vi "labview_code.vi"() -> ()   [LabVIEW 2025]
uses:
  Program Files (x86)/National Instruments/LabVIEW 2025/examples/Instrument IO/Serial/support/Serial - Settings.ctl
  Program Files (x86)/National Instruments/LabVIEW 2025/examples/Instrument IO/Serial/support/Serial - XON-XOFF Characters.ctl
  Program Files (x86)/National Instruments/LabVIEW 2025/examples/Instrument IO/Serial/support/Serial - ASCII Characters.ctl
  <vilib>/Utility/config.llb/Read Key (U32).vi
  <vilib>/Utility/config.llb/Read Key (String).vi
  <vilib>/Instr/_visa.llb/VISA Configure Serial Port (Instr).vi
  <vilib>/Utility/config.llb/NI_LVConfig.lvlib
panel:
  out "MSG from STM32 board 2":string
  in  "Termination Character 5":u8=10 format="%.0x"
  out "Updated baud rate":string
  out "read buffer 3":string
  in  "Stop 5":bool
  in  "Termination Character 4":u8=10 format="%.0x"
  in  "End Write on Termination Character? 4":bool=TRUE
  in  "XON/XOFF Characters 4":T1={"XON"=enum."DC1", "XOFF"=enum."DC3"}
  in  "Serial Settings 4":T3={"baud rate"=9600, "data bits"=8, "parity"=enum."None", "stop bits"=10, "flow control"=0} {"flow control" items=["None"=0, "XON/XOFF"=1, "RTS/CTS"=2, "DTR/DSR"=4]; "stop bits" items=["1.0"=10, "1.5"=15, "2.0"=20]; "data bits" min=5 max=8 step=1; "baud rate" items=["75"=75, "110"=110, "134"=134, "150"=150, "300"=300, "600"=600, "1200"=1200, "1800"=1800, "2400"=2400, "4800"=4800, "7200"=7200, "9600"=9600, "14400"=14400, "19200"=19200, "28800"=28800, "38400"=38400, "56000"=56000, "57600"=57600, "115200"=115200, "128000"=128000, "230400"=230400]}
  in  "End Read on Termination Character? 4":bool=TRUE
  in  "Stop 4":bool
  in  "Termination Character 3":u8=10 format="%.0x"
  in  "End Write on Termination Character? 3":bool=TRUE
  in  "XON/XOFF Characters 3":T1={"XON"=enum."DC1", "XOFF"=enum."DC3"}
  in  "Serial Settings 3":T3={"baud rate"=9600, "data bits"=8, "parity"=enum."None", "stop bits"=10, "flow control"=0} {"flow control" items=["None"=0, "XON/XOFF"=1, "RTS/CTS"=2, "DTR/DSR"=4]; "stop bits" items=["1.0"=10, "1.5"=15, "2.0"=20]; "data bits" min=5 max=8 step=1; "baud rate" items=["75"=75, "110"=110, "134"=134, "150"=150, "300"=300, "600"=600, "1200"=1200, "1800"=1800, "2400"=2400, "4800"=4800, "7200"=7200, "9600"=9600, "14400"=14400, "19200"=19200, "28800"=28800, "38400"=38400, "56000"=56000, "57600"=57600, "115200"=115200, "128000"=128000, "230400"=230400]}
  in  "End Read on Termination Character? 3":bool=TRUE
  out "read buffer 2":string
  in  "Stop 3":bool
  in  "Termination Character 2":u8=10 format="%.0x"
  in  "End Write on Termination Character? 2":bool=TRUE
  in  "XON/XOFF Characters 2":T1={"XON"=enum."DC1", "XOFF"=enum."DC3"}
  in  "Serial Settings 2":T3={"baud rate"=9600, "data bits"=8, "parity"=enum."None", "stop bits"=10, "flow control"=0} {"flow control" items=["None"=0, "XON/XOFF"=1, "RTS/CTS"=2, "DTR/DSR"=4]; "stop bits" items=["1.0"=10, "1.5"=15, "2.0"=20]; "data bits" min=5 max=8 step=1; "baud rate" items=["75"=75, "110"=110, "134"=134, "150"=150, "300"=300, "600"=600, "1200"=1200, "1800"=1800, "2400"=2400, "4800"=4800, "7200"=7200, "9600"=9600, "14400"=14400, "19200"=19200, "28800"=28800, "38400"=38400, "56000"=56000, "57600"=57600, "115200"=115200, "128000"=128000, "230400"=230400]}
  in  "End Read on Termination Character? 2":bool=TRUE
  out "Data Shift":string
  out "Handshake":string
  out "data out 2":string
  out "read buffer":string
  in  "Stop 2":bool
  in  "Termination Character":u8=10 format="%.0x"
  in  "End Write on Termination Character?":bool=TRUE
  in  "XON/XOFF Characters":T1={"XON"=enum."DC1", "XOFF"=enum."DC3"}
  in  "Serial Settings":T3={"baud rate"=9600, "data bits"=8, "parity"=enum."None", "stop bits"=10, "flow control"=0} {"flow control" items=["None"=0, "XON/XOFF"=1, "RTS/CTS"=2, "DTR/DSR"=4]; "stop bits" items=["1.0"=10, "1.5"=15, "2.0"=20]; "data bits" min=5 max=8 step=1; "baud rate" items=["75"=75, "110"=110, "134"=134, "150"=150, "300"=300, "600"=600, "1200"=1200, "1800"=1800, "2400"=2400, "4800"=4800, "7200"=7200, "9600"=9600, "14400"=14400, "19200"=19200, "28800"=28800, "38400"=38400, "56000"=56000, "57600"=57600, "115200"=115200, "128000"=128000, "230400"=230400]}
  in  "End Read on Termination Character?":bool=TRUE
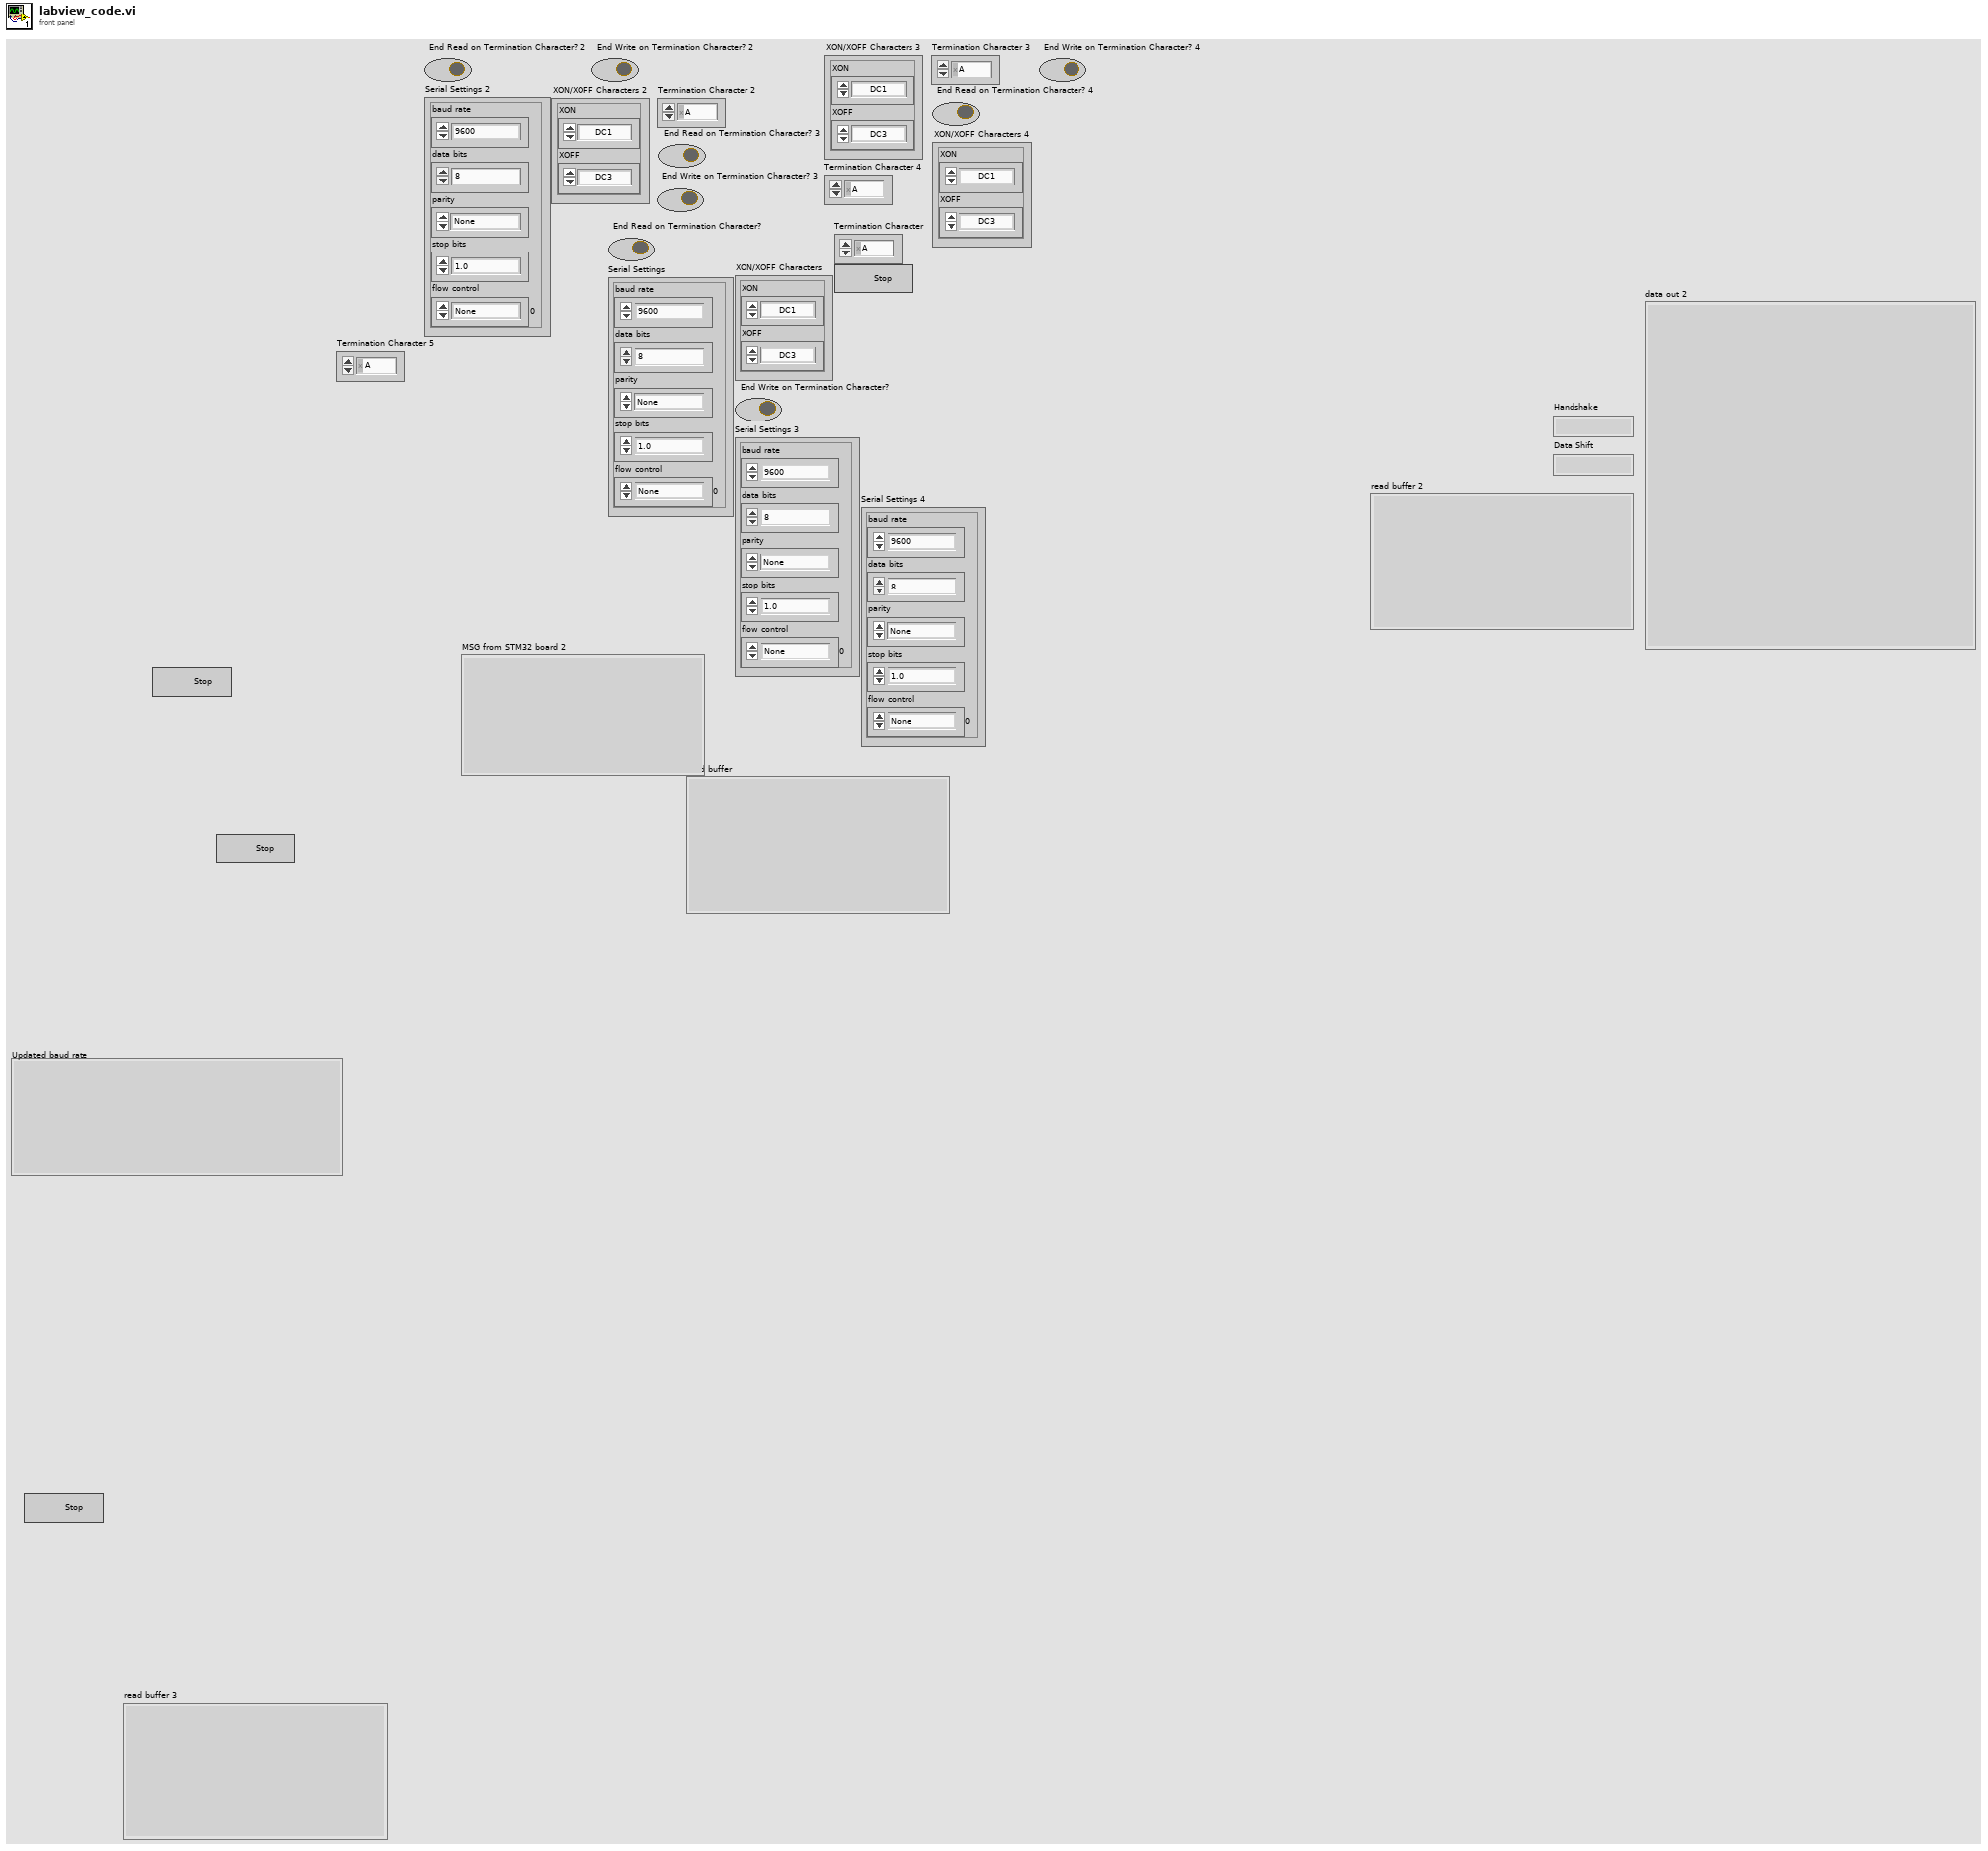
[diagram p1: front panel]
types:
  T1 = typedef "Serial - XON-XOFF Characters.ctl" = cluster{"XON":T2, "XOFF":T2}
  T2 = typedef "Serial - ASCII Characters.ctl" = enum16{"NUL", "SOH", "STX", "ETX", "EOT", "ENQ", "ACK", "BEL", "BS", "HT", "LF", "VT", "FF", "CR", "SO", "SI", "DLE", "DC1", "DC2", "DC3", "DC4", "NAK", "SYN", "ETB", "CAN", "EM", "SUB", "ESC", "FS", "GS", "RS", "US", "SP", "!", "\"", "#", "$", "%", "&", "'", "(", ")", "*", "+", ",", "- (-)", ".", "/", "0", "1", "2", "3", "4", "5", "6", "7", "8", "9", ":", ";", "<", "=", ">", "?", "@", "A", "B", "C", "D", "E", "F", "G", "H", "I", "J", "K", "L", "M", "N", "O", "P", "Q", "R", "S", "T", "U", "V", "W", "X", "Y", "Z", "[", "\\", "]", "^", "_", "`", "a", "b", "c", "d", "e", "f", "g", "h", "i", "j", "k", "l", "m", "n", "o", "p", "q", "r", "s", "t", "u", "v", "w", "x", "y", "z", "{", "|", "}", "~"}
  T3 = typedef "Serial - Settings.ctl" = cluster{"baud rate":u32, "data bits":u16, "parity":enum16{"None", "Odd", "Even", "Mark", "Space"}, "stop bits":u16, "flow control":u16}
  T4 = enum16{"Standard", "Buffered", "CRLF", "Immediate"}
  T5 = typedef "NI_LVConfig.lvlib/Config Data RefNum.ctl" = refnum<k1>
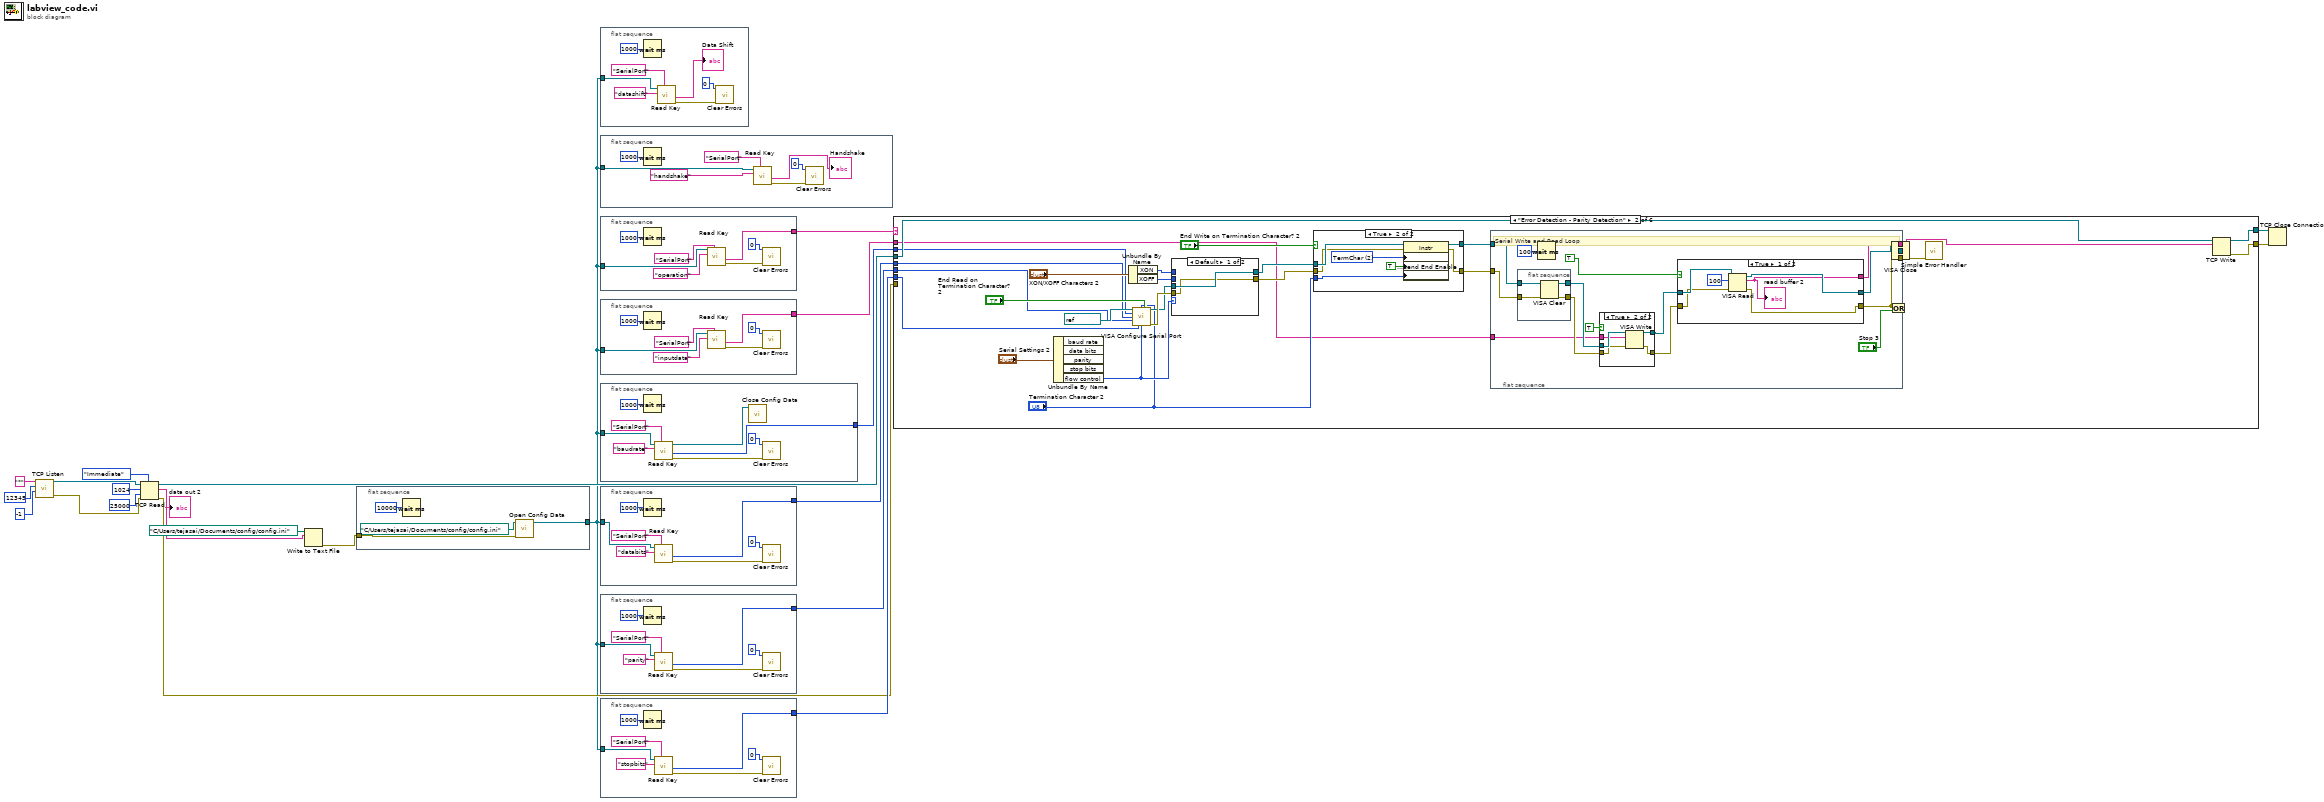
[diagram p0: block diagram]
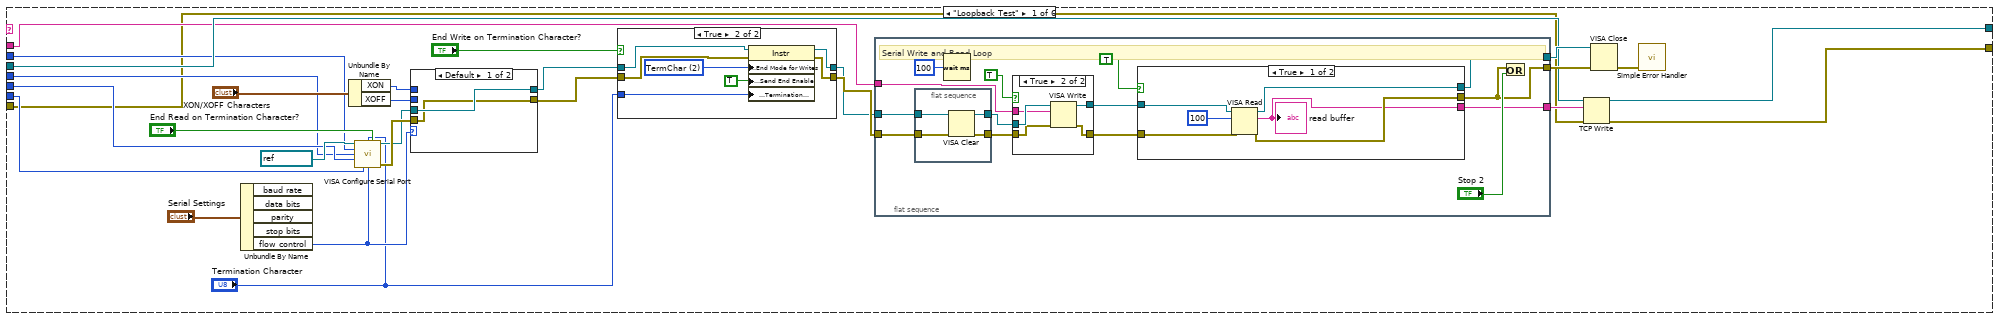
[diagram p2: hidden frame]
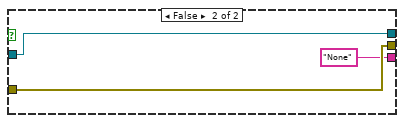
[diagram p3: hidden frame]
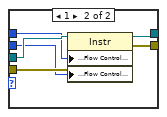
[diagram p6: hidden frame]
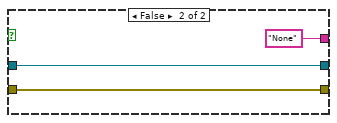
[diagram p8: hidden frame]
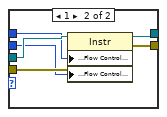
[diagram p10: hidden frame]
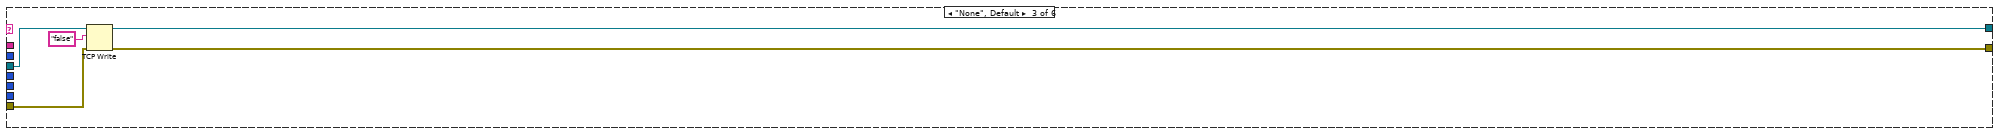
[diagram p11: hidden frame]
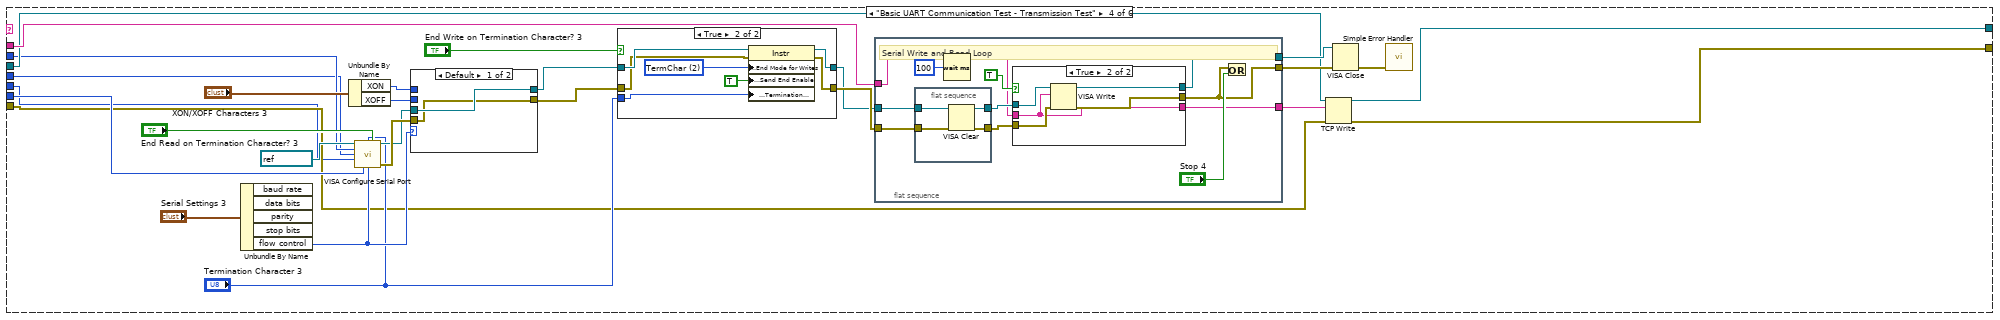
[diagram p12: hidden frame]
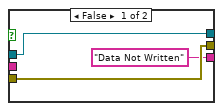
[diagram p13: hidden frame]
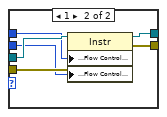
[diagram p15: hidden frame]
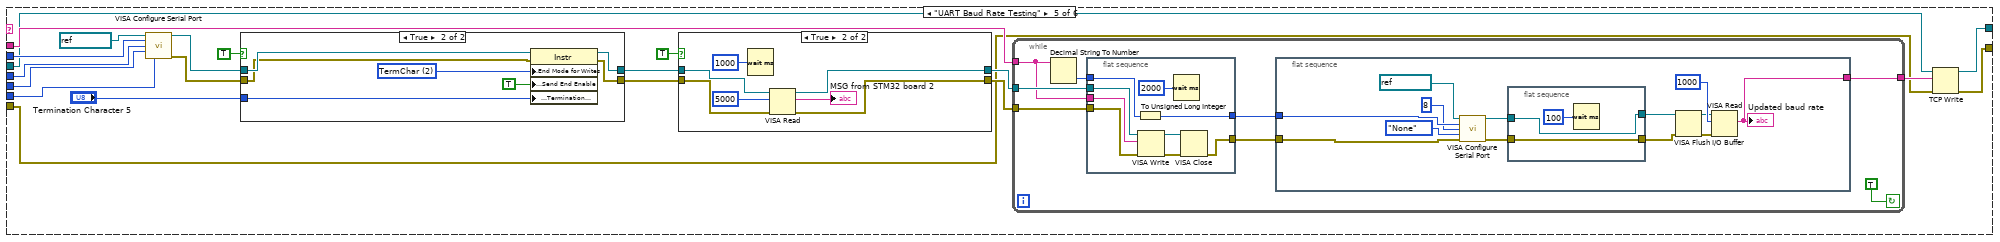
[diagram p16: hidden frame]
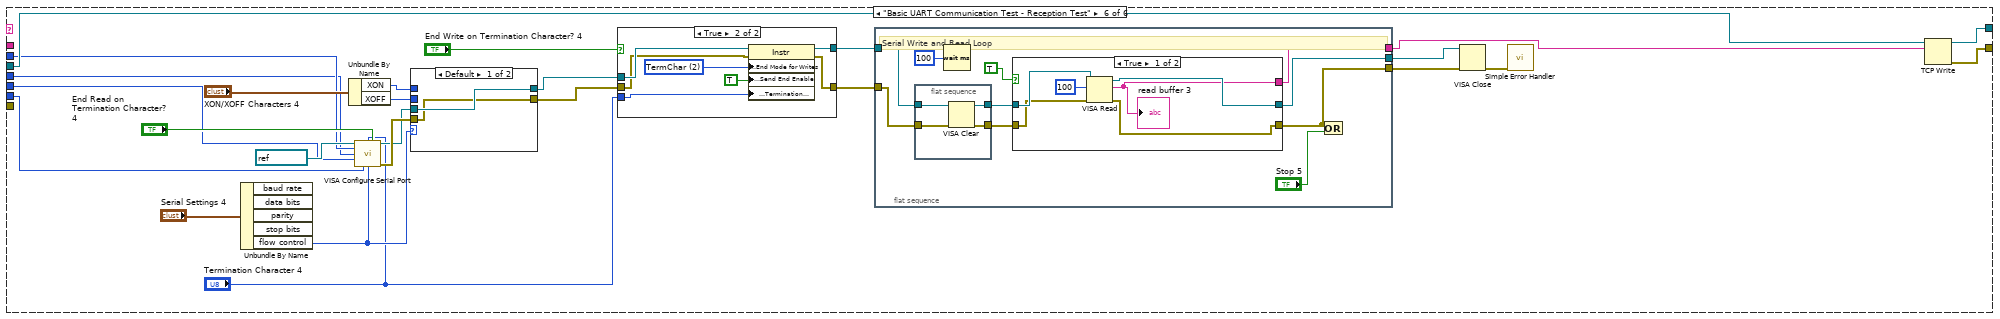
[diagram p19: hidden frame]
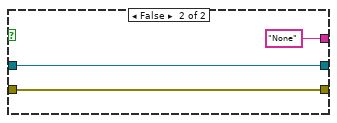
[diagram p20: hidden frame]
diagram:
  n1 = call <vilib>:"TCP Listen.vi"("timeout ms (wait forever: -1)"=-1, "port"=u16 12345, "service name"="*") -> ("error out"=w5:errorcluster, "connection ID"=w6:refnum<k5>)  [unwired: 4 in, 3 out]
  n2 = TCP Read(connection ID=w6, bytes to read=1024, error in (no error)=w5, 7:T4."Immediate" ("mode (standard)"), 9:25000 ("timeout ms (25000)")) -> (connection ID out=w4:refnum<k5>, data out=w7:string, error out=w3:errorcluster)
  "data out 2" <- w7
  n3 = Write to Text File(file (use dialog)=path "C:/Users/tejasai/Documents/config/config.ini", text=w7) -> (error out=w21:errorcluster)  [unwired: 2 in, 2 out]
  n4 = flat-sequence {
    tunnel: w21 -> [w25]
    tunnel: [w24] -> w2
    frame #0 {
      n5 = Wait (ms)(milliseconds to wait=u32 10000) -> ()  [unwired: 1 out]
      n6 = call <vilib>:"Open Config Data.vi"("error in (no error)"=w25, "configuration file path"=path "C:/Users/tejasai/Documents/config/config.ini") -> ("refnum"=w24:T5)  [unwired: 7 in, 2 out]
    }
  }
  n7 = flat-sequence {
    tunnel: w2 -> [w30]
    frame #0 {
      n8 = Wait (ms)(milliseconds to wait=u32 1000) -> ()  [unwired: 1 out]
      n9 = call-poly <vilib>:"Read Key.vi"("section"="SerialPort", "key"="datashift", "refnum"=w30) -> ("error out"=w28:errorcluster, "value"=→"Data Shift":string)  [unwired: 5 in, 2 out]
      n10 = call <vilib>:"Clear Errors.vi"("error in (no error)"=w28, "specific error code to clear (0: all)"=0) -> ()  [unwired: 4 in, 2 out]
    }
  }
  n11 = flat-sequence {
    tunnel: w2 -> [w37]
    frame #0 {
      n12 = Wait (ms)(milliseconds to wait=u32 1000) -> ()  [unwired: 1 out]
      n13 = call-poly <vilib>:"Read Key.vi"("section"="SerialPort", "key"="handshake", "refnum"=w37) -> ("error out"=w35:errorcluster, "value"=→"Handshake":string)  [unwired: 5 in, 2 out]
      n14 = call <vilib>:"Clear Errors.vi"("error in (no error)"=w35, "specific error code to clear (0: all)"=0) -> ()  [unwired: 4 in, 2 out]
    }
  }
  n15 = flat-sequence {
    tunnel: [w45] -> w19
    tunnel: w2 -> [w44]
    frame #0 {
      n16 = Wait (ms)(milliseconds to wait=u32 1000) -> ()  [unwired: 1 out]
      n17 = call-poly <vilib>:"Read Key.vi"("section"="SerialPort", "key"="operation", "refnum"=w44) -> ("error out"=w42:errorcluster, "value"=w45:string)  [unwired: 5 in, 2 out]
      n18 = call <vilib>:"Clear Errors.vi"("error in (no error)"=w42, "specific error code to clear (0: all)"=0) -> ()  [unwired: 4 in, 2 out]
    }
  }
  n19 = flat-sequence {
    tunnel: [w52] -> w18
    tunnel: w2 -> [w51]
    frame #0 {
      n20 = Wait (ms)(milliseconds to wait=u32 1000) -> ()  [unwired: 1 out]
      n21 = call-poly <vilib>:"Read Key.vi"("section"="SerialPort", "key"="inputdata", "refnum"=w51) -> ("error out"=w49:errorcluster, "value"=w52:string)  [unwired: 5 in, 2 out]
      n22 = call <vilib>:"Clear Errors.vi"("error in (no error)"=w49, "specific error code to clear (0: all)"=0) -> ()  [unwired: 4 in, 2 out]
    }
  }
  n23 = flat-sequence {
    tunnel: [w59] -> w17
    tunnel: w2 -> [w58]
    frame #0 {
      n24 = Wait (ms)(milliseconds to wait=u32 1000) -> ()  [unwired: 1 out]
      n25 = call-poly <vilib>:"Read Key.vi"("section"="SerialPort", "key"="baudrate", "refnum"=w58) -> ("error out"=w56:errorcluster, "value"=w59:u32, "refnum out"=w62:T5)  [unwired: 5 in, 1 out]
      n26 = call <vilib>:"Close Config Data.vi"("refnum"=w62) -> ()  [unwired: 9 in, 2 out]
      n27 = call <vilib>:"Clear Errors.vi"("error in (no error)"=w56, "specific error code to clear (0: all)"=0) -> ()  [unwired: 4 in, 2 out]
    }
  }
  n28 = flat-sequence {
    tunnel: [w67] -> w16
    tunnel: w2 -> [w66]
    frame #0 {
      n29 = Wait (ms)(milliseconds to wait=u32 1000) -> ()  [unwired: 1 out]
      n30 = call-poly <vilib>:"Read Key.vi"("section"="SerialPort", "key"="databits", "refnum"=w66) -> ("error out"=w64:errorcluster, "value"=w67:u32)  [unwired: 5 in, 2 out]
      n31 = call <vilib>:"Clear Errors.vi"("error in (no error)"=w64, "specific error code to clear (0: all)"=0) -> ()  [unwired: 4 in, 2 out]
    }
  }
  n32 = flat-sequence {
    tunnel: [w74] -> w15
    tunnel: w2 -> [w73]
    frame #0 {
      n33 = Wait (ms)(milliseconds to wait=u32 1000) -> ()  [unwired: 1 out]
      n34 = call-poly <vilib>:"Read Key.vi"("section"="SerialPort", "key"="parity", "refnum"=w73) -> ("error out"=w71:errorcluster, "value"=w74:u32)  [unwired: 5 in, 2 out]
      n35 = call <vilib>:"Clear Errors.vi"("error in (no error)"=w71, "specific error code to clear (0: all)"=0) -> ()  [unwired: 4 in, 2 out]
    }
  }
  n36 = flat-sequence {
    tunnel: [w81] -> w14
    tunnel: w2 -> [w80]
    frame #0 {
      n37 = Wait (ms)(milliseconds to wait=u32 1000) -> ()  [unwired: 1 out]
      n38 = call-poly <vilib>:"Read Key.vi"("section"="SerialPort", "key"="stopbits", "refnum"=w80) -> ("error out"=w78:errorcluster, "value"=w81:u32)  [unwired: 5 in, 2 out]
      n39 = call <vilib>:"Clear Errors.vi"("error in (no error)"=w78, "specific error code to clear (0: all)"=0) -> ()  [unwired: 4 in, 2 out]
    }
  }
  n40 = case shown="\"Error Detection - Parity Detection\"" w19 {
    tunnel: w4 -> [w93 w170 w243 w249 w317 w389]
    tunnel: w3 -> [w84 _ w242 w250 w316 _]
    tunnel: [w91 w169 w245 w254 w315 w391] -> w22
    tunnel: w18 -> [w89 w163 _ w252 w319 _]
    tunnel: w17 -> [w88 w164 _ w248 w323 w388]
    tunnel: w16 -> [w85 w166 _ w247 w322 w387]
    tunnel: w15 -> [w87 w167 _ w246 w321 w386]
    tunnel: w14 -> [w86 w165 _ w251 w320 w385]
    tunnel: [w90 w168 w244 w253 w314 w390] -> w1
    frame "Loopback Test" {
      n41 = Unbundle By Name("Serial Settings") -> ("flow control"=w103:u16)  [unwired: 4 out]
      n42 = Unbundle By Name("XON/XOFF Characters") -> ("XON"=w102:T2, "XOFF"=w101:T2)
      n43 = call-poly "VISA Configure Serial Port"("VISA resource name"=refnum<visa-resource-name> "COM5", "termination char\n(0xA = '\\n' = LF)"="Termination Character", "Enable Termination\nChar (T)"="End Read on Termination Character?", "baud rate (9600)"=w88, "data bits (8)"=w85, "parity (0:none)"=w87, "stop bits (10: 1 bit)"=w86, "flow control (0:none)"=w103) -> ("VISA resource name out"=w109:refnum<visa-resource-name>, "error out"=w110:errorcluster)  [unwired: 2 in, 4 out]
      n44 = case shown="Default" w103 {
        tunnel: [w155 w162] -> w100
        tunnel: [w156 w161] -> w98
        tunnel: w110 -> [w155 w160]
        tunnel: w109 -> [w156 w159]
        tunnel: w102 -> [_ w158]
        tunnel: w101 -> [_ w157]
        frame Default {
        }
        frame 1 {
          n45 = property class="Instr"(reference=w159, error in=w160, "Serial Settings:Flow Control XON Character"=w158, "Serial Settings:Flow Control XOFF Character"=w157) -> (reference out=w161:refnum<visa-resource-name>, error out=w162:errorcluster)
        }
      }
      n46 = case shown="True" "End Write on Termination Character?" {
        tunnel: w98 -> [w146 w154]
        tunnel: w100 -> [w147 w153]
        tunnel: [w146 w152] -> w97
        tunnel: [w147 w151] -> w99
        tunnel: "Termination Character" -> [_ w149]
        frame False {
        }
        frame True {
          w150 = u16 2 items=["None", "LastBit", "TermChar", "Break"] ("Serial Settings:Serial End Mode for Writes")
          n47 = property class="Instr"(reference=w154, error in=w153, "Serial Settings:End Mode for Writes"=w150, "Message Based Settings:Send End Enable"=TRUE, "Message Based Settings:Termination Character"=w149) -> (reference out=w152:refnum<visa-resource-name>, error out=w151:errorcluster)
        }
      }
      n48 = flat-sequence {
        tunnel: w99 -> [w122]
        tunnel: [w116] -> w105
        tunnel: w97 -> [w123]
        tunnel: [w117] -> w104
        tunnel: w89 -> [w119]
        tunnel: [w115] -> w92
        frame #0 {
          # "Serial Write and Read Loop"
          n49 = flat-sequence {
            tunnel: w123 -> [w138]
            tunnel: w122 -> [w137]
            tunnel: [w136] -> w120
            tunnel: [w135] -> w121
            frame #0 {
              n50 = VISA Clear(VISA resource name=w138, error in (no error)=w137) -> (VISA resource name out=w136:refnum<visa-resource-name>, error out=w135:errorcluster)
            }
          }
          n51 = Wait (ms)(milliseconds to wait=u32 100) -> ()  [unwired: 1 out]
          n52 = case shown="True" TRUE {
            tunnel: w120 -> [w140 w145]
            tunnel: w121 -> [w139 w144]
            tunnel: [w140 w143] -> w114
            tunnel: [w139 w142] -> w113
            tunnel: w119 -> [_ w141]
            frame False {
            }
            frame True {
              n53 = VISA Write(VISA resource name=w145, write buffer=w141, error in (no error)=w144) -> (VISA resource name out=w143:refnum<visa-resource-name>, error out=w142:errorcluster)  [unwired: 1 out]
            }
          }
          n54 = case shown="True" TRUE {
            tunnel: [w129 w134] -> w117
            tunnel: w114 -> [w131 w134]
            tunnel: [w128 w133] -> w116
            tunnel: w113 -> [w130 w133]
            tunnel: [w127 "None"] -> w115
            frame True {
              n55 = VISA Read(VISA resource name=w131, byte count=u32 100, error in (no error)=w130) -> (VISA resource name out=w129:refnum<visa-resource-name>, read buffer=w127:string, error out=w128:errorcluster)  [unwired: 1 out]
              "read buffer" <- w127
            }
            frame False {
            }
          }
          n56 = Or(x=w116, y="Stop 2") -> ()  [unwired: 1 out]
        }
      }
      n57 = TCP Write(connection ID=w93, data in=w92, error in (no error)=w84) -> (connection ID out=w91:refnum<k5>, error out=w90:errorcluster)  [unwired: 1 in, 1 out]
      n58 = VISA Close(VISA resource name=w104, error in (no error)=w105) -> (error out=w106:errorcluster)
      n59 = call <vilib>:"Simple Error Handler.vi"("error in (no error)"=w106) -> ()  [unwired: 1 in, 8 out]
    }
    frame "Error Detection - Parity Detection" {
      n60 = Unbundle By Name("Serial Settings 2") -> ("flow control"=w181:u16)  [unwired: 4 out]
      n61 = Unbundle By Name("XON/XOFF Characters 2") -> ("XON"=w180:T2, "XOFF"=w179:T2)
      n62 = call-poly "VISA Configure Serial Port"("VISA resource name"=refnum<visa-resource-name> "COM4", "termination char\n(0xA = '\\n' = LF)"="Termination Character 2", "Enable Termination\nChar (T)"="End Read on Termination Character? 2", "baud rate (9600)"=w164, "data bits (8)"=w166, "parity (0:none)"=w167, "stop bits (10: 1 bit)"=w165, "flow control (0:none)"=w181) -> ("VISA resource name out"=w187:refnum<visa-resource-name>, "error out"=w188:errorcluster)  [unwired: 2 in, 4 out]
      n63 = case shown="Default" w181 {
        tunnel: [w233 w240] -> w178
        tunnel: [w234 w239] -> w176
        tunnel: w188 -> [w233 w238]
        tunnel: w187 -> [w234 w237]
        tunnel: w180 -> [_ w236]
        tunnel: w179 -> [_ w235]
        frame Default {
        }
        frame 1 {
          n64 = property class="Instr"(reference=w237, error in=w238, "Serial Settings:Flow Control XON Character"=w236, "Serial Settings:Flow Control XOFF Character"=w235) -> (reference out=w239:refnum<visa-resource-name>, error out=w240:errorcluster)
        }
      }
      n65 = case shown="True" "End Write on Termination Character? 2" {
        tunnel: w176 -> [w224 w232]
        tunnel: w178 -> [w225 w231]
        tunnel: [w224 w230] -> w175
        tunnel: [w225 w229] -> w177
        tunnel: "Termination Character 2" -> [_ w227]
        frame False {
        }
        frame True {
          w228 = u16 2 items=["None", "LastBit", "TermChar", "Break"] ("Serial Settings:Serial End Mode for Writes")
          n66 = property class="Instr"(reference=w232, error in=w231, "Serial Settings:End Mode for Writes"=w228, "Message Based Settings:Send End Enable"=TRUE, "Message Based Settings:Termination Character"=w227) -> (reference out=w230:refnum<visa-resource-name>, error out=w229:errorcluster)
        }
      }
      n67 = flat-sequence {
        tunnel: w177 -> [w201]
        tunnel: [w198] -> w183
        tunnel: w175 -> [w202]
        tunnel: [w199] -> w182
        tunnel: [w197] -> w171
        tunnel: w163 -> [w191]
        frame #0 {
          # "Serial Write and Read Loop"
          n68 = flat-sequence {
            tunnel: w202 -> [w223]
            tunnel: w201 -> [w222]
            tunnel: [w221] -> w195
            tunnel: [w220] -> w194
            frame #0 {
              n69 = VISA Clear(VISA resource name=w223, error in (no error)=w222) -> (VISA resource name out=w221:refnum<visa-resource-name>, error out=w220:errorcluster)
            }
          }
          n70 = Wait (ms)(milliseconds to wait=u32 100) -> ()  [unwired: 1 out]
          n71 = case shown="True" TRUE {
            tunnel: w195 -> [w205 w210]
            tunnel: w194 -> [w204 w209]
            tunnel: [w205 w208] -> w193
            tunnel: [w204 w207] -> w192
            tunnel: w191 -> [_ w206]
            frame False {
            }
            frame True {
              n72 = VISA Write(VISA resource name=w210, write buffer=w206, error in (no error)=w209) -> (VISA resource name out=w208:refnum<visa-resource-name>, error out=w207:errorcluster)  [unwired: 1 out]
            }
          }
          n73 = case shown="True" TRUE {
            tunnel: [w214 w219] -> w199
            tunnel: w193 -> [w216 w219]
            tunnel: [w213 w218] -> w198
            tunnel: w192 -> [w215 w218]
            tunnel: [w212 "None"] -> w197
            frame True {
              n74 = VISA Read(VISA resource name=w216, byte count=u32 100, error in (no error)=w215) -> (VISA resource name out=w214:refnum<visa-resource-name>, read buffer=w212:string, error out=w213:errorcluster)  [unwired: 1 out]
              "read buffer 2" <- w212
            }
            frame False {
            }
          }
          n75 = Or(x=w198, y="Stop 3") -> ()  [unwired: 1 out]
        }
      }
      n76 = VISA Close(VISA resource name=w182, error in (no error)=w183) -> (error out=w184:errorcluster)
      n77 = call <vilib>:"Simple Error Handler.vi"("error in (no error)"=w184) -> ()  [unwired: 1 in, 8 out]
      n78 = TCP Write(connection ID=w170, data in=w171) -> (connection ID out=w169:refnum<k5>, error out=w168:errorcluster)  [unwired: 2 in, 1 out]
    }
    frame "None", Default {
      n79 = TCP Write(connection ID=w243, data in="false", error in (no error)=w242) -> (connection ID out=w245:refnum<k5>, error out=w244:errorcluster)  [unwired: 1 in, 1 out]
    }
    frame "Basic UART Communication Test - Transmission Test" {
      n80 = Unbundle By Name("Serial Settings 3") -> ("flow control"=w265:u16)  [unwired: 4 out]
      n81 = Unbundle By Name("XON/XOFF Characters 3") -> ("XON"=w264:T2, "XOFF"=w263:T2)
      n82 = call-poly "VISA Configure Serial Port"("VISA resource name"=refnum<visa-resource-name> "COM7", "termination char\n(0xA = '\\n' = LF)"="Termination Character 3", "Enable Termination\nChar (T)"="End Read on Termination Character? 3", "baud rate (9600)"=w248, "data bits (8)"=w247, "parity (0:none)"=w246, "stop bits (10: 1 bit)"=w251, "flow control (0:none)"=w265) -> ("VISA resource name out"=w271:refnum<visa-resource-name>, "error out"=w272:errorcluster)  [unwired: 2 in, 4 out]
      n83 = case shown="Default" w265 {
        tunnel: [w306 w313] -> w262
        tunnel: [w307 w312] -> w260
        tunnel: w272 -> [w306 w311]
        tunnel: w271 -> [w307 w310]
        tunnel: w264 -> [_ w309]
        tunnel: w263 -> [_ w308]
        frame Default {
        }
        frame 1 {
          n84 = property class="Instr"(reference=w310, error in=w311, "Serial Settings:Flow Control XON Character"=w309, "Serial Settings:Flow Control XOFF Character"=w308) -> (reference out=w312:refnum<visa-resource-name>, error out=w313:errorcluster)
        }
      }
      n85 = case shown="True" "End Write on Termination Character? 3" {
        tunnel: w260 -> [w297 w305]
        tunnel: w262 -> [w298 w304]
        tunnel: [w297 w303] -> w259
        tunnel: [w298 w302] -> w261
        tunnel: "Termination Character 3" -> [_ w300]
        frame False {
        }
        frame True {
          w301 = u16 2 items=["None", "LastBit", "TermChar", "Break"] ("Serial Settings:Serial End Mode for Writes")
          n86 = property class="Instr"(reference=w305, error in=w304, "Serial Settings:End Mode for Writes"=w301, "Message Based Settings:Send End Enable"=TRUE, "Message Based Settings:Termination Character"=w300) -> (reference out=w303:refnum<visa-resource-name>, error out=w302:errorcluster)
        }
      }
      n87 = flat-sequence {
        tunnel: w261 -> [w281]
        tunnel: [w275] -> w267
        tunnel: w259 -> [w282]
        tunnel: [w276] -> w266
        tunnel: w252 -> [w278]
        tunnel: [w274] -> w255
        frame #0 {
          # "Serial Write and Read Loop"
          n88 = flat-sequence {
            tunnel: w282 -> [w288]
            tunnel: w281 -> [w287]
            tunnel: [w286] -> w279
            tunnel: [w285] -> w280
            frame #0 {
              n89 = VISA Clear(VISA resource name=w288, error in (no error)=w287) -> (VISA resource name out=w286:refnum<visa-resource-name>, error out=w285:errorcluster)
            }
          }
          n90 = Wait (ms)(milliseconds to wait=u32 100) -> ()  [unwired: 1 out]
          n91 = case shown="True" TRUE {
            tunnel: w279 -> [w291 w296]
            tunnel: w280 -> [w290 w295]
            tunnel: [w291 w294] -> w276
            tunnel: [w290 w293] -> w275
            tunnel: w278 -> [_ w292]
            tunnel: ["Data Not Written" w292] -> w274
            frame False {
            }
            frame True {
              n92 = VISA Write(VISA resource name=w296, write buffer=w292, error in (no error)=w295) -> (VISA resource name out=w294:refnum<visa-resource-name>, error out=w293:errorcluster)  [unwired: 1 out]
            }
          }
          n93 = Or(x=w275, y="Stop 4") -> ()  [unwired: 1 out]
        }
      }
      n94 = TCP Write(connection ID=w249, data in=w255, error in (no error)=w250) -> (connection ID out=w254:refnum<k5>, error out=w253:errorcluster)  [unwired: 1 in, 1 out]
      n95 = VISA Close(VISA resource name=w266, error in (no error)=w267) -> (error out=w268:errorcluster)
      n96 = call <vilib>:"Simple Error Handler.vi"("error in (no error)"=w268) -> ()  [unwired: 1 in, 8 out]
    }
    frame "UART Baud Rate Testing" {
      n97 = call-poly "VISA Configure Serial Port"("VISA resource name"=refnum<visa-resource-name> "COM7", "baud rate (9600)"=w323, "data bits (8)"=w322, "parity (0:none)"=w321, "stop bits (10: 1 bit)"=w320) -> ("VISA resource name out"=w332:refnum<visa-resource-name>, "error out"=w331:errorcluster)  [unwired: 9 in]
      n98 = case shown="True" TRUE {
        tunnel: w332 -> [w343 w351]
        tunnel: w331 -> [w344 w350]
        tunnel: [w343 w349] -> w328
        tunnel: [w344 w348] -> w327
        tunnel: "Termination Character 5" -> [_ w346]
        frame False {
        }
        frame True {
          w347 = u16 2 items=["None", "LastBit", "TermChar", "Break"] ("Serial Settings:Serial End Mode for Writes")
          n99 = property class="Instr"(reference=w351, error in=w350, "Serial Settings:End Mode for Writes"=w347, "Message Based Settings:Send End Enable"=TRUE, "Message Based Settings:Termination Character"=w346) -> (reference out=w349:refnum<visa-resource-name>, error out=w348:errorcluster)
        }
      }
      n100 = case shown="True" TRUE {
        tunnel: w328 -> [w335 w339]
        tunnel: w327 -> [w334 w338]
        tunnel: [w335 w337] -> w325
        tunnel: [w334 w336] -> w324
        frame False {
        }
        frame True {
          n101 = Wait (ms)(milliseconds to wait=u32 1000) -> ()  [unwired: 1 out]
          n102 = VISA Read(VISA resource name=w339, byte count=u32 5000, error in (no error)=w338) -> (VISA resource name out=w337:refnum<visa-resource-name>, read buffer=→"MSG from STM32 board 2":string, error out=w336:errorcluster)  [unwired: 1 out]
        }
      }
      n103 = while {
        tunnel: w325 -> [w359]
        tunnel: w324 -> [w358]
        tunnel: w319 -> [w354]
        tunnel: [w352] -> w318
        stop <- TRUE continue-if-true
        n104 = Decimal String To Number(string=w354) -> (number=w353:i32)  [unwired: 2 in, 1 out]
        n105 = flat-sequence {
          tunnel: w359 -> [w383]
          tunnel: w358 -> [w382]
          tunnel: [w381] -> w356
          tunnel: [w378] -> w355
          tunnel: w354 -> [w377]
          tunnel: w353 -> [w376]
          frame #0 {
            n106 = To Unsigned Long Integer(number=w376) -> (unsigned 32bit integer=w381:u32)
            n107 = VISA Write(VISA resource name=w383, write buffer=w377, error in (no error)=w382) -> (VISA resource name out=w380:refnum<visa-resource-name>, error out=w379:errorcluster)  [unwired: 1 out]
            n108 = Wait (ms)(milliseconds to wait=u32 2000) -> ()  [unwired: 1 out]
            n109 = VISA Close(VISA resource name=w380, error in (no error)=w379) -> (error out=w378:errorcluster)
          }
        }
        n110 = flat-sequence {
          tunnel: w356 -> [w370]
          tunnel: w355 -> [w367]
          tunnel: [w360] -> w352
          frame #0 {
            n111 = call-poly "VISA Configure Serial Port"("VISA resource name"=refnum<visa-resource-name> "COM4", "baud rate (9600)"=w370, "data bits (8)"=u16 8, "parity (0:none)"=enum16{"None", "Odd", "Even", "Mark", "Space"}."None", "error in (no error)"=w367) -> ("VISA resource name out"=w366:refnum<visa-resource-name>, "error out"=w363:errorcluster)  [unwired: 9 in]
            n112 = flat-sequence {
              tunnel: w366 -> [w374]
              tunnel: [w374] -> w365
              tunnel: [w373] -> w364
              tunnel: w363 -> [w373]
              frame #0 {
                n113 = Wait (ms)(milliseconds to wait=u32 100) -> ()  [unwired: 1 out]
              }
            }
            n114 = VISA Flush I/O Buffer(VISA resource name=w365, error in (no error)=w364) -> (VISA resource name out=w362:refnum<visa-resource-name>, error out=w361:errorcluster)  [unwired: 1 in]
            n115 = VISA Read(VISA resource name=w362, byte count=u32 1000, error in (no error)=w361) -> (read buffer=w360:string)  [unwired: 3 out]
            "Updated baud rate" <- w360
          }
        }
      }
      n116 = TCP Write(connection ID=w317, data in=w318, error in (no error)=w316) -> (connection ID out=w315:refnum<k5>, error out=w314:errorcluster)  [unwired: 1 in, 1 out]
    }
    frame "Basic UART Communication Test - Reception Test" {
      n117 = Unbundle By Name("Serial Settings 4") -> ("flow control"=w402:u16)  [unwired: 4 out]
      n118 = Unbundle By Name("XON/XOFF Characters 4") -> ("XON"=w401:T2, "XOFF"=w400:T2)
      n119 = call-poly "VISA Configure Serial Port"("VISA resource name"=refnum<visa-resource-name> "COM7", "termination char\n(0xA = '\\n' = LF)"="Termination Character 4", "Enable Termination\nChar (T)"="End Read on Termination Character? 4", "baud rate (9600)"=w388, "data bits (8)"=w387, "parity (0:none)"=w386, "stop bits (10: 1 bit)"=w385, "flow control (0:none)"=w402) -> ("VISA resource name out"=w408:refnum<visa-resource-name>, "error out"=w409:errorcluster)  [unwired: 2 in, 4 out]
      n120 = case shown="Default" w402 {
        tunnel: [w443 w450] -> w399
        tunnel: [w444 w449] -> w397
        tunnel: w409 -> [w443 w448]
        tunnel: w408 -> [w444 w447]
        tunnel: w401 -> [_ w446]
        tunnel: w400 -> [_ w445]
        frame Default {
        }
        frame 1 {
          n121 = property class="Instr"(reference=w447, error in=w448, "Serial Settings:Flow Control XON Character"=w446, "Serial Settings:Flow Control XOFF Character"=w445) -> (reference out=w449:refnum<visa-resource-name>, error out=w450:errorcluster)
        }
      }
      n122 = case shown="True" "End Write on Termination Character? 4" {
        tunnel: w397 -> [w434 w442]
        tunnel: w399 -> [w435 w441]
        tunnel: [w434 w440] -> w396
        tunnel: [w435 w439] -> w398
        tunnel: "Termination Character 4" -> [_ w437]
        frame False {
        }
        frame True {
          w438 = u16 2 items=["None", "LastBit", "TermChar", "Break"] ("Serial Settings:Serial End Mode for Writes")
          n123 = property class="Instr"(reference=w442, error in=w441, "Serial Settings:End Mode for Writes"=w438, "Message Based Settings:Send End Enable"=TRUE, "Message Based Settings:Termination Character"=w437) -> (reference out=w440:refnum<visa-resource-name>, error out=w439:errorcluster)
        }
      }
      n124 = flat-sequence {
        tunnel: w398 -> [w418]
        tunnel: [w415] -> w404
        tunnel: w396 -> [w419]
        tunnel: [w416] -> w403
        tunnel: [w414] -> w392
        frame #0 {
          # "Serial Write and Read Loop"
          n125 = flat-sequence {
            tunnel: w419 -> [w433]
            tunnel: w418 -> [w432]
            tunnel: [w431] -> w412
            tunnel: [w430] -> w411
            frame #0 {
              n126 = VISA Clear(VISA resource name=w433, error in (no error)=w432) -> (VISA resource name out=w431:refnum<visa-resource-name>, error out=w430:errorcluster)
            }
          }
          n127 = Wait (ms)(milliseconds to wait=u32 100) -> ()  [unwired: 1 out]
          n128 = case shown="True" TRUE {
            tunnel: [w424 w429] -> w416
            tunnel: w412 -> [w426 w429]
            tunnel: [w423 w428] -> w415
            tunnel: w411 -> [w425 w428]
            tunnel: [w422 "None"] -> w414
            frame True {
              n129 = VISA Read(VISA resource name=w426, byte count=u32 100, error in (no error)=w425) -> (VISA resource name out=w424:refnum<visa-resource-name>, read buffer=w422:string, error out=w423:errorcluster)  [unwired: 1 out]
              "read buffer 3" <- w422
            }
            frame False {
            }
          }
          n130 = Or(x=w415, y="Stop 5") -> ()  [unwired: 1 out]
        }
      }
      n131 = VISA Close(VISA resource name=w403, error in (no error)=w404) -> (error out=w405:errorcluster)
      n132 = call <vilib>:"Simple Error Handler.vi"("error in (no error)"=w405) -> ()  [unwired: 1 in, 8 out]
      n133 = TCP Write(connection ID=w389, data in=w392) -> (connection ID out=w391:refnum<k5>, error out=w390:errorcluster)  [unwired: 2 in, 1 out]
    }
  }
  n134 = TCP Close Connection(connection ID=w22, error in (no error)=w1) -> ()  [unwired: 1 in, 2 out]
